vi "ADCS.Port.Create.vi"(10 "Enable Stream":bool, 11 "CAN port":string) -> (3 "CAN port out":string)   [LabVIEW 2019, in "Diagnostics Addon Engine.lvlib"]
uses:
  Diagnostics Addon Engine.lvlib
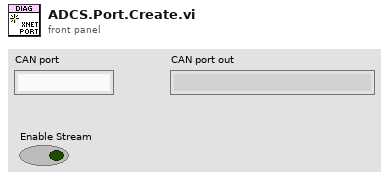
[diagram p1: front panel]
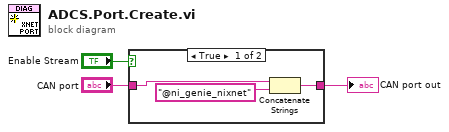
[diagram p0: block diagram]
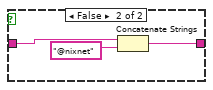
[diagram p2: hidden frame]
diagram:
  n1 = case shown="True" "Enable Stream" {
    tunnel: "CAN port" -> [w6 w9]
    tunnel: [w5 w8] -> w2
    frame True {
      n2 = Concatenate Strings(w6, "@ni_genie_nixnet" ("string")) -> (w5:string)
    }
    frame False {
      n3 = Concatenate Strings(w9, "@nixnet" ("string")) -> (w8:string)
    }
  }
  "CAN port out" <- w2
